vi "CreateNewBoard_FixedSize.vi"(8 "error in (no error)":errorcluster, 10 "BoardSize":u16) -> (0 "error out":errorcluster, 2 "Board out":refnum<class "Board.lvclass">)   [LabVIEW 2015, in "TronviewGame.lvlib" / "GameBuilder.lvclass"]
uses:
  GameBuilder.lvclass
  Board/Board.lvclass
  Board/BoardSize.ctl
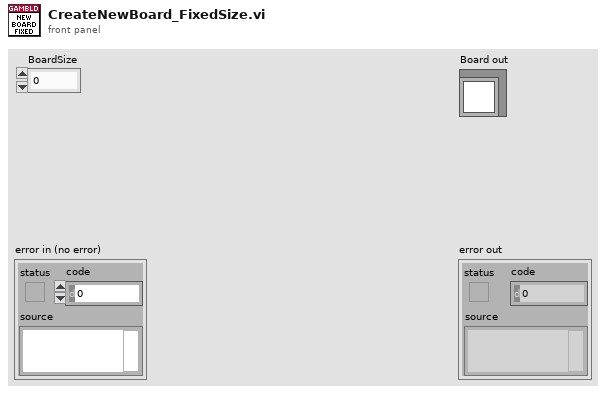
[diagram p1: front panel]
types:
  T1 = typedef "TronviewGame.lvlib/Board.lvclass/BoardSize.ctl" = cluster{"Columns":u16, "Rows":u16}
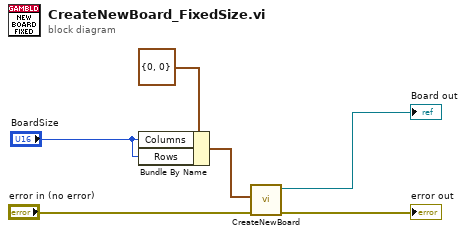
[diagram p0: block diagram]
diagram:
  n1 = Bundle By Name(cluster=T1 {"Columns"=0, "Rows"=0} ("Size"), "Columns"="BoardSize", "Rows"="BoardSize") -> (w5:T1)
  n2 = call "CreateNewBoard.vi"("error in (no error)"="error in (no error)", "Size"=w5) -> ("error out"=→"error out":errorcluster, "Board out"=→"Board out":refnum<class "Board.lvclass">)  [unwired: 8 in]
